vi "MessageName.vi"() -> (2 "MessageName":string)   [LabVIEW 2020, in "TcpClientHello.lvlib"]
uses:
  TcpClientHello.lvlib
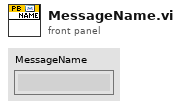
[diagram p1: front panel]
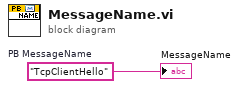
[diagram p0: block diagram]
diagram:
  w1 = "TcpClientHello"  # PB MessageName
  "MessageName" <- w1
